vi "pp2_log_toString_trial.vi"(11 "Trial in":T1={"Trial Type Number"=1, "Trial Type"=enum."GO", "Trial Weight"=100, "Shock (mA)"=0.3, "Duration (ms)"=0.25, "Sound Type"=enum."04 FM Sweep", "Stim P1"=4000.0, "Stim P2"=0.0, "Stim P3"=0.0, "Stim P4"=2000.0} {"Shock (mA)" min=-1.0 max=5.0; "Trial Weight" step=1; "Duration (ms)" min=0.0 max=1.0; "Trial Type Number" min=1 max=256 step=1}) -> (3 "spreadsheet string":string)   [LabVIEW 2013]
uses:
  pp2_CTL_Trial.ctl
  pp2_CTL_TrialType.ctl
  labolabo2/waveforms/WFTypes.ctl
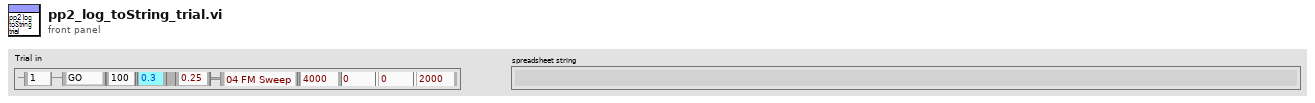
[diagram p1: front panel]
types:
  T1 = typedef "pp2_CTL_Trial.ctl" = cluster{"Trial Type Number":i16, "Trial Type":T2, "Trial Weight":u32, "Shock (mA)":dbl, "Duration (ms)":dbl, "Sound Type":T3, "Stim P1":dbl, "Stim P2":dbl, "Stim P3":dbl, "Stim P4":dbl}
  T2 = typedef "pp2_CTL_TrialType.ctl" = enum16{"OFF", "GO", "NOGO", "TEST"}
  T3 = typedef "WFTypes.ctl" = enum16{"00 NULL", "01 DC", "02 Noise", "03 Pure Tone", "04 FM Sweep"}
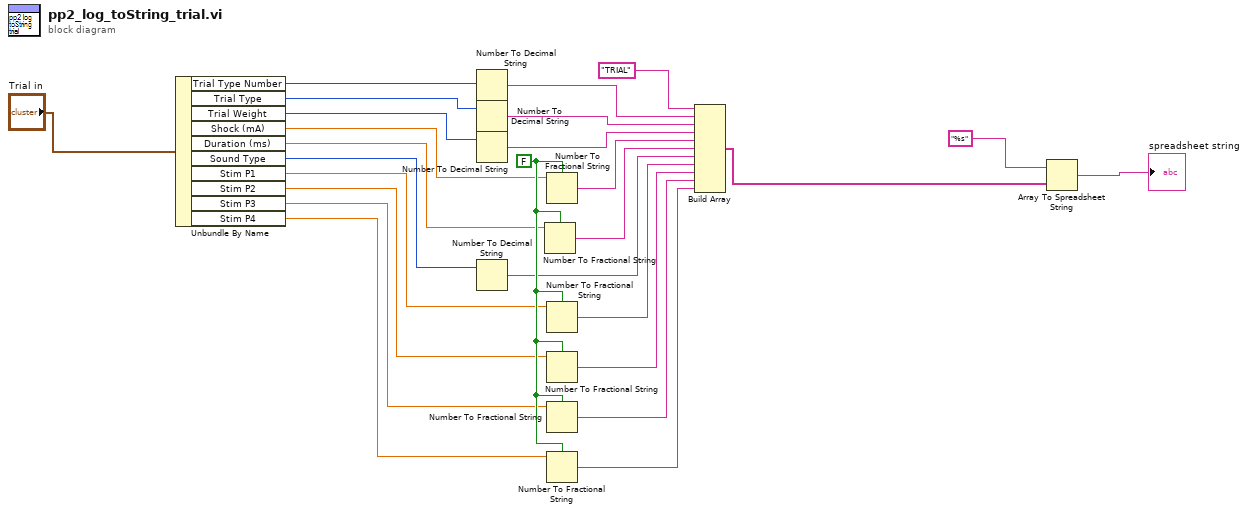
[diagram p0: block diagram]
diagram:
  w15 = FALSE
  n1 = Unbundle By Name("Trial in") -> ("Trial Type Number"=w19:i16, "Trial Type"=w18:T2, "Trial Weight"=w17:u32, "Shock (mA)"=w7:dbl, "Duration (ms)"=w6:dbl, "Sound Type"=w16:T3, "Stim P1"=w5:dbl, "Stim P2"=w4:dbl, "Stim P3"=w3:dbl, "Stim P4"=w2:dbl)
  n2 = Number To Decimal String(number=w19) -> (decimal integer string=w21:string)  [unwired: 1 in]
  n3 = Number To Decimal String(number=w18) -> (decimal integer string=w26:string)  [unwired: 1 in]
  n4 = Number To Decimal String(number=w17) -> (decimal integer string=w25:string)  [unwired: 1 in]
  n5 = Number To Decimal String(number=w16) -> (decimal integer string=w12:string)  [unwired: 1 in]
  n6 = Number To Fractional String(use system decimal point (T)=w15, number=w6) -> (F-format string=w13:string)  [unwired: 2 in]
  n7 = Number To Fractional String(use system decimal point (T)=w15, number=w7) -> (F-format string=w14:string)  [unwired: 2 in]
  n8 = Number To Fractional String(use system decimal point (T)=w15, number=w5) -> (F-format string=w11:string)  [unwired: 2 in]
  n9 = Number To Fractional String(use system decimal point (T)=w15, number=w4) -> (F-format string=w10:string)  [unwired: 2 in]
  n10 = Number To Fractional String(use system decimal point (T)=w15, number=w3) -> (F-format string=w9:string)  [unwired: 2 in]
  n11 = Number To Fractional String(use system decimal point (T)=w15, number=w2) -> (F-format string=w8:string)  [unwired: 2 in]
  n12 = Build Array("TRIAL" ("element"), w21, w26, w25, w14, w13, w12, w11, w10, w9, w8) -> (w23:string[])
  n13 = Array To Spreadsheet String(array=w23, 3:"%s" ("format string")) -> (spreadsheet string=→"spreadsheet string":string)  [unwired: 1 in]
